vi "Find Controllers.vi"(8 "error in (no error)":errorcluster) -> (0 "error out":errorcluster, 2 "Num of Controllers":i32, 3 "Names":string[](array[string]))   [LabVIEW 2020]
uses:
  libximc.lvlib
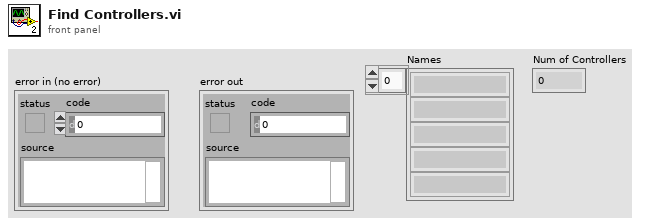
[diagram p1: front panel]
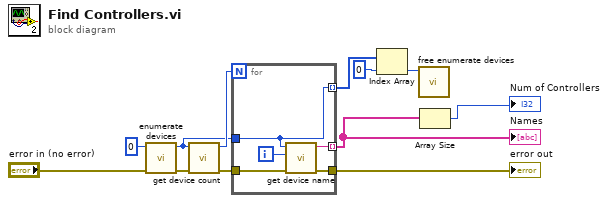
[diagram p0: block diagram]
diagram:
  n1 = call "enumerate devices.vi"("error in (no error)"="error in (no error)", "enumerate_flags"=0 ("probe_devices")) -> ("error out"=w8:errorcluster, "function return"=w6:u32)  [unwired: 8 in]
  n2 = call "get device count.vi"("error in (no error)"=w8, "device_enumeration"=w6) -> ("error out"=w9:errorcluster, "function return"=w10:i32)  [unwired: 8 in]
  n3 = for {
    N: w10 -> [_]
    tunnel: [w17] -> w7
    tunnel: [w16] -> w2 mode=indexing
    tunnel: w6 -> [w13]
    tunnel: w9 -> [w14]
    tunnel: [w13] -> w5 mode=indexing
    i -> [w15]
    n4 = call "get device name.vi"("error in (no error)"=w14, "device_index"=w15, "device_enumeration"=w13) -> ("error out"=w17:errorcluster, "function return"=w16:string)  [unwired: 7 in]
  }
  "error out" <- w7
  "Names" <- w2
  n5 = Index Array(array=w5, index=0 ("probe_devices")) -> (element=w3:u32)
  n6 = call "free enumerate devices.vi"("device_enumeration"=w3) -> ()  [unwired: 9 in, 2 out]
  n7 = Array Size(array=w2) -> (size(s)=→"Num of Controllers":i32)
